vi "Volt Meter.vi"() -> ()   [LabVIEW 2010]
panel:
  out "Voltage":dbl
  in  "Data Acquisition Interval (s)":dbl min=0.01 max=60.0
  in  "stop":bool
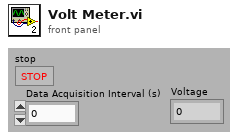
[diagram p1: front panel]
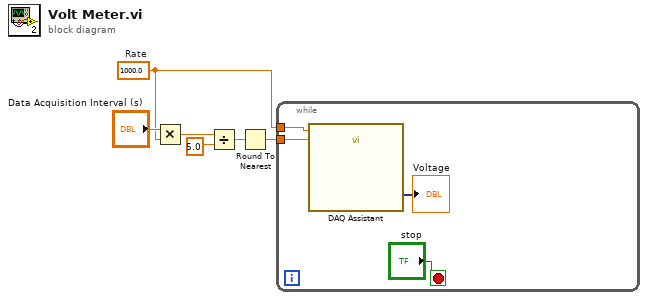
[diagram p0: block diagram]
diagram:
  w1 = 1000.0  # Rate
  n1 = Multiply(x="Data Acquisition Interval (s)", y=w1) -> (x*y=w5:dbl)
  n2 = Divide(x=w5, y=5.0) -> (x/y=w3:dbl)
  n3 = Round To Nearest(number=w3) -> (nearest integer value=w2:dbl)
  n4 = while {
    tunnel: w2 -> [w9]
    tunnel: w1 -> [w8]
    stop <- "stop" stop-if-true
    n5 = call "DAQ Assistant"("rate"=w8, "number of samples"=w9) -> ("data"=→"Voltage":dynamicdata)  [unwired: 15 in, 2 out]
  }
